vi "CS POLARIS BME DG.ProcCases.vi"(0 "i ref in":refnum<vi>, 1 "selector":string, 2 "Data":T1, 3 "call cluster":T2={"Object"="", "Selector"="", "CallType"=enum."synchronous", "Async Object"="", "Async Selector"="", "Data Descriptor"="", "Data"=[], "Error #"=0, "Expire"=0}, 5 "error in (no error)":errorcluster) -> (14 "i ref out":refnum<vi>, 17 "answer cluster":T2={"Object"="", "Selector"="", "CallType"=enum."synchronous", "Async Object"="", "Async Selector"="", "Data Descriptor"="", "Data"=[], "Error #"=0, "Expire"=0}, 19 "error out":errorcluster)   [LabVIEW 2009, in "CS POLARIS BME DG.lvlib"]
doc: "This method is called by a process from within the default case in the event loop. The methods of a class that are linked to events will be called from THIS method. Add your code here."
uses:
  CS POLARIS BME DG.lvlib
  CSCore/CSSystem/CoreDefs/CoreDefs.call_type.ctl
  CSCore/BaseProcess/BaseProcess.descriptor string definition.ctl
  CSCore/CSSystem/CoreDefs/CoreDefs.rawDataType.ctl
  CSCore/CSSystem/CoreLib/CoreLib.byte array 2 string.vi
  DG Classes/BME_DG_System/ControlLevel.ctl
  DG Classes/BME_DG_System/BME_DG_System.lvclass
  CSCore/CSSystem/CoreLib/CoreLib.byte array 2 int.vi
  DG Classes/BME_DG_Chnl/BME_DG_Chnl.lvclass
  CSCore/CSSystem/CoreLib/CoreLib.double 2 byte array.vi
  CSCore/CSSystem/CoreLib/CoreLib.string 2 byte array.vi
  CSCore/CSSystem/CoreLib/CoreLib.lvlib
  CSCore/BaseProcess/BaseProcess.lvlib
  CSApplicationBaseClasses/DeviceBase/DeviceBase.lvlib
  lib.lib/UtilityLib/UtilityLib.lvlib
  lib.lib/DimLVEvent/LVDimInterface/LVDimInterface.lvlib
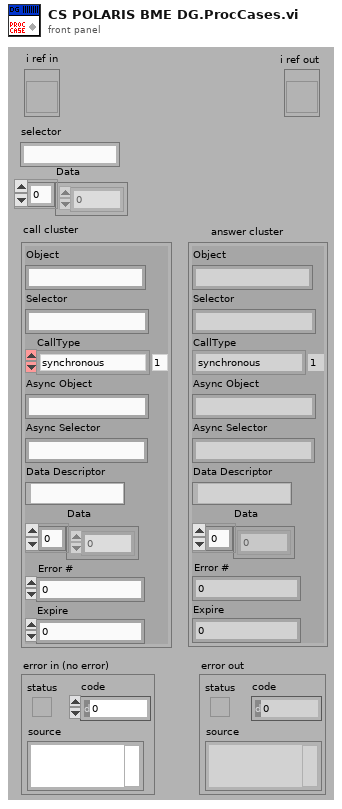
[diagram p1: front panel]
types:
  T1 = typedef "CoreDefs.rawDataType.ctl" = i8[]
  T2 = typedef "CoreDefs.call_type.ctl" = cluster{"Object":string, "Selector":string, "CallType":enum16{"simple", "synchronous", "asynchronous"}, "Async Object":string, "Async Selector":string, "Data Descriptor":T3, "Data":T1, "Error #":i32, "Expire":u32}
  T3 = typedef "BaseProcess.lvlib/BaseProcess.descriptor string definition.ctl" = string
  T4 = typedef "POLARIS BME DG.lvlib/BME_DG_System.lvclass/ControlLevel.ctl" = enum16{"Simple", "Expert", "Unknown"}
  T5 = typedef "POLARIS BME DG.lvlib/Chnl Settings Complete.ctl" = cluster{"Channel Name":string, "ChnParameter":T6, "DelayFormula":string, "OutputModulo":i32, "Go and Done Signal":T7, "G08_Chnl_Settings":T9}
  T6 = typedef "POLARIS BME DG.lvlib/ChnlSettings.ctl" = cluster{" Delay (µs)":dbl, "On?":bool, "PositiveVoltage?":bool, "50OhmTerminated? ":bool, "25OhmOutput?":bool}
  T7 = typedef "POLARIS BME DG.lvlib/Go_Done_Chnl_Settings.ctl" = cluster{"Go Signal":T8, "Done Signal":u32}
  T8 = typedef "POLARIS BME DG.lvlib/GoSignalBits.ctl" = u32
  T9 = typedef "POLARIS BME DG.lvlib/SG08_Chnl_Settings.ctl" = cluster{"Pulse Width (µs)":dbl, "Output Offset":u32, "Disconnect (E,F)":bool, "Onto MsBus (E,F)":bool, "Input Positive (E,F)":bool}
  T10 = typedef "CS POLARIS BME DG.lvlib/CS POLARIS BME DG.i attribute.ctl" = cluster{"DIMLockedBy":i32, "DG_System":refnum<queue>, "UpdateTasks":refnum<queue>, "SaveEachParamChng":bool, "SaveAtShutdown":bool, "DIMSecTillComShot":i32}
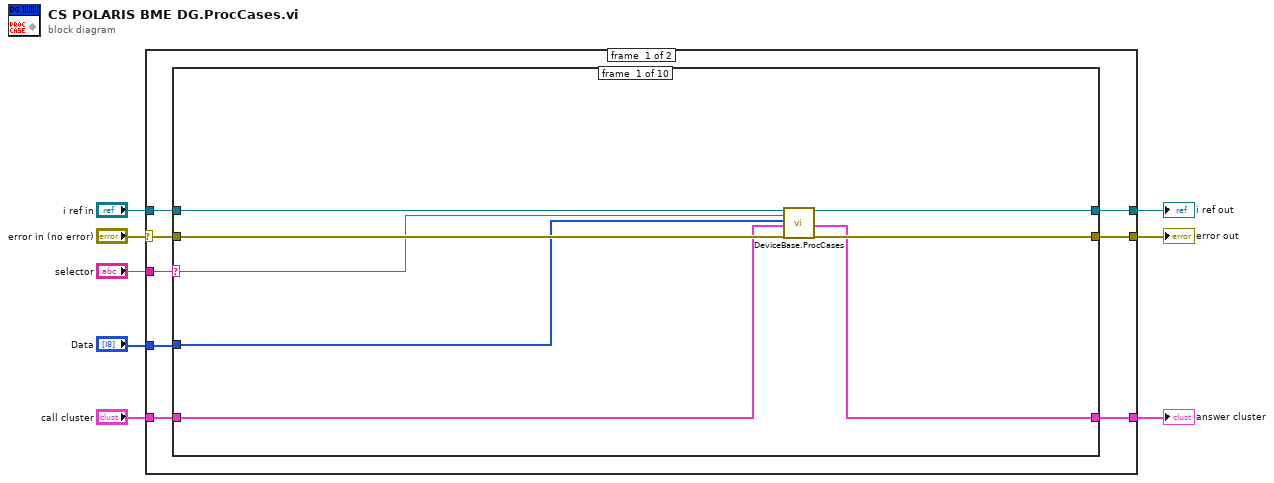
[diagram p0: block diagram]
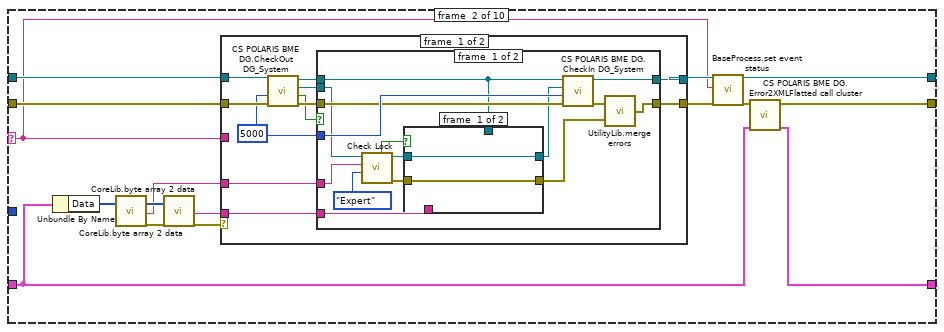
[diagram p2: hidden frame]
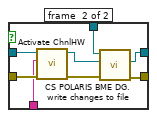
[diagram p3: hidden frame]
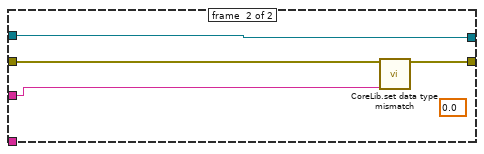
[diagram p5: hidden frame]
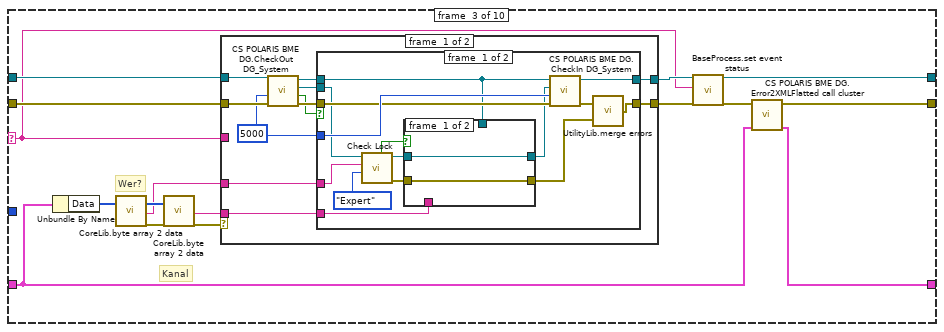
[diagram p6: hidden frame]
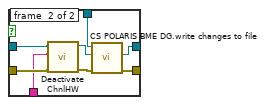
[diagram p7: hidden frame]
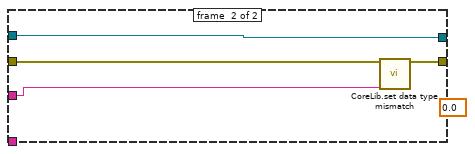
[diagram p9: hidden frame]
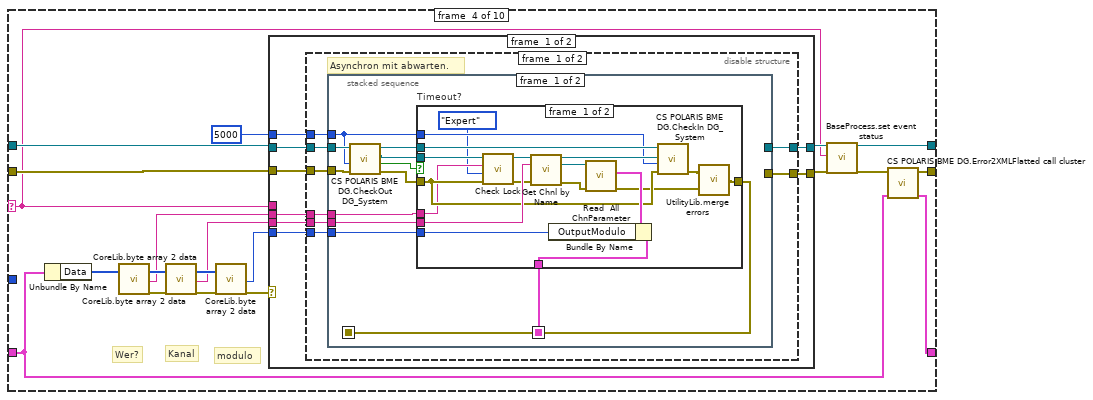
[diagram p10: hidden frame]
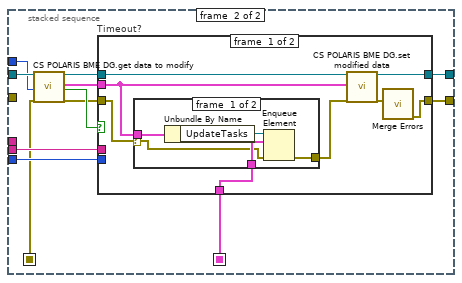
[diagram p12: hidden frame]
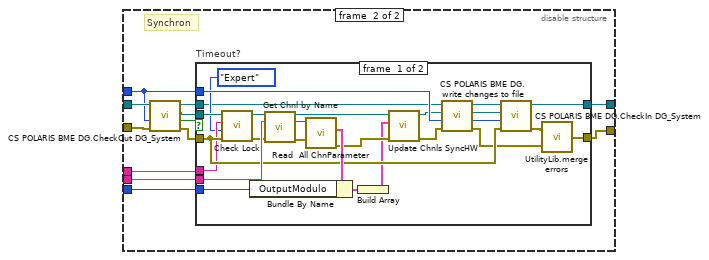
[diagram p15: hidden frame]
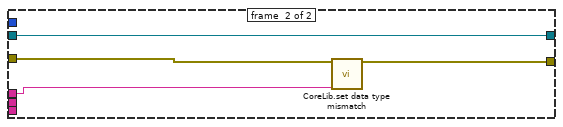
[diagram p17: hidden frame]
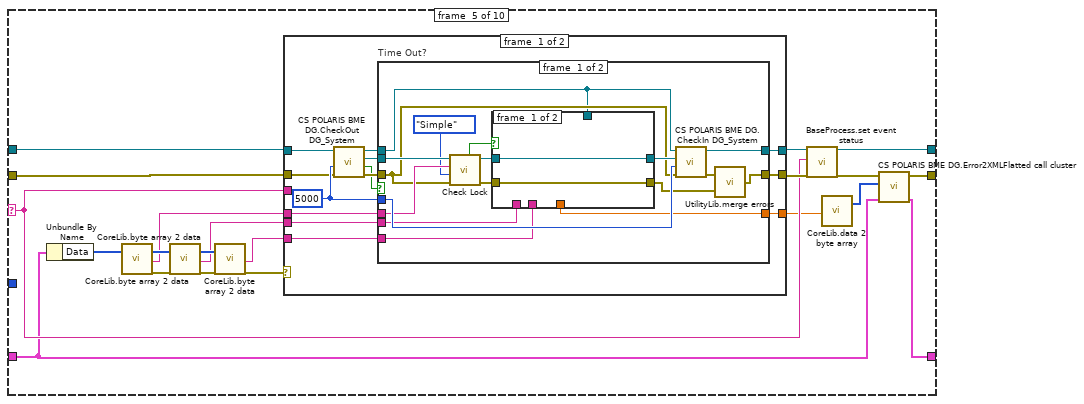
[diagram p18: hidden frame]
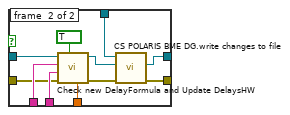
[diagram p19: hidden frame]
diagram:
  n1 = case shown="No Error" "error in (no error)" {
    selector: "error in (no error)" -> [w9 w596]
    tunnel: "selector" -> [w16 _]
    tunnel: [w15 w597] -> w7
    tunnel: "Data" -> [w14 _]
    tunnel: "call cluster" -> [w13 w597]
    tunnel: "i ref in" -> [w12 w598]
    tunnel: [w11 w598] -> w3
    tunnel: [w10 w596] -> w2
    frame #0 {
      n2 = case shown="\"SetDelayFormula\"" w16 {
        selector: w16 -> [w19 w36 w94 w156 w295 w361 w412 w462 w517 w562]
        tunnel: w14 -> [w17 _ _ _ _ _ _ _ _ _]
        tunnel: w12 -> [w18 w40 w98 w160 w299 w365 w416 w466 w521 w565]
        tunnel: [w24 w35 w93 w155 w294 w360 w411 w461 w516 w561] -> w11
        tunnel: w13 -> [w20 w30 w88 w146 w286 w351 w406 w455 w511 w558]
        tunnel: [w21 w29 w87 w147 w285 w350 w405 w454 w510 w557] -> w15
        tunnel: w9 -> [w23 w39 w97 w159 w298 w364 w415 w465 w520 w555]
        tunnel: [w22 w31 w89 w148 w287 w352 w407 w456 w512 w559] -> w10
        frame #0 {
          # "In the default case, always call the ProcCase method of the parent class"
          n3 = call "DeviceBase.ProcCases.vi"("i ref in"=w18, "selector"=w19, "Data"=w17, "call cluster"=w20, "error in (no error)"=w23) -> ("i ref out"=w24:refnum<vi>, "answer cluster"=w21:T2, "error out"=w22:errorcluster)  [unwired: 12 in]
        }
        frame #1 {
          # "This is just an example. On how to use this VI. The names of the selector should be identical to the name of the corresponding event. Inside the false case, place the method you want to call."
          n4 = Unbundle By Name(w30) -> ("Data"=w27:T1)
          n5 = call-poly "CoreLib.byte array 2 data.vi"("byteArray"=w27) -> ("byteArray out"=w28:T1, "string"=w25:string, "error out"=w26:errorcluster)  [unwired: 16 in]
          n6 = call-poly "CoreLib.byte array 2 data.vi"("byteArray"=w28, "error in (no error)"=w26) -> ("string"=w33:string, "error out"=w34:errorcluster)  [unwired: 15 in, 1 out]
          n7 = case shown="No Error" w34 {
            tunnel: [w46 w82] -> w38
            tunnel: w40 -> [w51 w82]
            tunnel: w39 -> [w50 w81]
            tunnel: [w44 w80] -> w37
            tunnel: w36 -> [_ w79]
            tunnel: w33 -> [w42 _]
            tunnel: w25 -> [w41 _]
            frame #0 {
              w43 = 5000 ("timeout in ms (-1)")
              n8 = call "CS POLARIS BME DG.CheckOut DG_System.vi"("error IO"=w50, "timeout in ms (-1)"=w43, "i ref in"=w51) -> ("error out"=w48:errorcluster, "Q timed out"=w47:bool, "BME_DG_System out"=w49:refnum<class "BME_DG_System.lvclass">, "i ref out"=w45:refnum<vi>)  [unwired: 5 in]
              n9 = case shown="False" w47 {
                tunnel: w49 -> [w57 _]
                tunnel: w48 -> [w64 w78]
                tunnel: [w62 w78] -> w44
                tunnel: [w66 w77] -> w46
                tunnel: w45 -> [w52 w77]
                tunnel: w43 -> [w65 _]
                tunnel: w42 -> [w54 _]
                tunnel: w41 -> [w53 _]
                frame #0 {
                  n10 = call-dynamic "Check Lock.vi"("Control level"=ControlLevel."Expert", "Name"=w53, "BME_DG_System in"=w57) -> ("error out"=w61:errorcluster, "BME_DG_System out"=w60:refnum<class "BME_DG_System.lvclass">, "Ok?"=w58:bool)  [unwired: 4 in, 2 out]
                  n11 = case shown="True" w58 {
                    tunnel: [w68 w70] -> w55
                    tunnel: w54 -> [_ w74]
                    tunnel: [w67 w69] -> w56
                    tunnel: w61 -> [w67 w75]
                    tunnel: w60 -> [w68 w76]
                    tunnel: w52 -> [_ w73]
                    frame #0 {
                    }
                    frame #1 {
                      n12 = call "Activate ChnlHW.vi"("error in (no error)"=w75, "ChnlName"=w74, "BME_DG_System in"=w76) -> ("error out"=w71:errorcluster, "BME_DG_System out"=w72:refnum<class "BME_DG_System.lvclass">)  [unwired: 7 in]
                      n13 = call "CS POLARIS BME DG.write changes to file.vi"("error in"=w71, "BME_DG_System in"=w72, "i ref in"=w73) -> ("error in"=w69:errorcluster, "BME_DG_System out"=w70:refnum<class "BME_DG_System.lvclass">)  [unwired: 5 in, 1 out]
                    }
                  }
                  n14 = call "CS POLARIS BME DG.CheckIn DG_System.vi"("error in"=w64, "timeout in ms (-1)"=w65, "BME_DG_System"=w55, "i ref in"=w52) -> ("error in"=w63:errorcluster, "i ref out"=w66:refnum<vi>)  [unwired: 5 in]
                  n15 = call "UtilityLib.merge errors.vi"("error2 (no error)"=w56, "error1 (no error)"=w63) -> ("error out"=w62:errorcluster)
                }
                frame #1 {
                }
              }
            }
            frame #1 {
              (unwired) 0.0
              n16 = call "CoreLib.set data type mismatch.vi"("error in (no error)"=w81, "error source"=w79) -> ("error out"=w80:errorcluster)  [unwired: 17 in]
            }
          }
          n17 = call "BaseProcess.set event status.vi"("i ref in"=w38, "EventStatus"=w36, "error in (no error)"=w37) -> ("i ref out"=w35:refnum<vi>, "error out"=w32:errorcluster)  [unwired: 14 in, 1 out]
          n18 = call "CS POLARIS BME DG.Error2XMLFlatted call cluster.vi"("call cluster in"=w30, "error in"=w32) -> ("call cluster out"=w29:T2, "error out"=w31:errorcluster)  [unwired: 8 in]
        }
        frame #2 {
          # "Kanal"
          # "Wer?"
          # "This is just an example. On how to use this VI. The names of the selector should be identical to the name of the corresponding event. Inside the false case, place the method you want to call."
          n19 = Unbundle By Name(w88) -> ("Data"=w85:T1)
          n20 = call-poly "CoreLib.byte array 2 data.vi"("byteArray"=w85) -> ("byteArray out"=w86:T1, "string"=w83:string, "error out"=w84:errorcluster)  [unwired: 16 in]
          n21 = call-poly "CoreLib.byte array 2 data.vi"("byteArray"=w86, "error in (no error)"=w84) -> ("string"=w91:string, "error out"=w92:errorcluster)  [unwired: 15 in, 1 out]
          n22 = case shown="No Error" w92 {
            tunnel: [w104 w140] -> w96
            tunnel: w98 -> [w109 w140]
            tunnel: w97 -> [w108 w139]
            tunnel: [w102 w138] -> w95
            tunnel: w94 -> [_ w137]
            tunnel: w91 -> [w100 _]
            tunnel: w83 -> [w99 _]
            frame #0 {
              w101 = 5000 ("timeout in ms (-1)")
              n23 = call "CS POLARIS BME DG.CheckOut DG_System.vi"("error IO"=w108, "timeout in ms (-1)"=w101, "i ref in"=w109) -> ("error out"=w106:errorcluster, "Q timed out"=w105:bool, "BME_DG_System out"=w107:refnum<class "BME_DG_System.lvclass">, "i ref out"=w103:refnum<vi>)  [unwired: 5 in]
              n24 = case shown="False" w105 {
                tunnel: w107 -> [w115 _]
                tunnel: w106 -> [w122 w136]
                tunnel: [w120 w136] -> w102
                tunnel: [w124 w135] -> w104
                tunnel: w103 -> [w110 w135]
                tunnel: w101 -> [w123 _]
                tunnel: w100 -> [w112 _]
                tunnel: w99 -> [w111 _]
                frame #0 {
                  n25 = call-dynamic "Check Lock.vi"("Control level"=ControlLevel."Expert", "Name"=w111, "BME_DG_System in"=w115) -> ("error out"=w119:errorcluster, "BME_DG_System out"=w118:refnum<class "BME_DG_System.lvclass">, "Ok?"=w116:bool)  [unwired: 4 in, 2 out]
                  n26 = case shown="True" w116 {
                    tunnel: [w126 w128] -> w113
                    tunnel: w112 -> [_ w132]
                    tunnel: [w125 w127] -> w114
                    tunnel: w119 -> [w125 w133]
                    tunnel: w118 -> [w126 w134]
                    tunnel: w110 -> [_ w131]
                    frame #0 {
                    }
                    frame #1 {
                      n27 = call "Deactivate ChnlHW.vi"("error in (no error)"=w133, "ChnlName"=w132, "BME_DG_System in"=w134) -> ("error out"=w129:errorcluster, "BME_DG_System out"=w130:refnum<class "BME_DG_System.lvclass">)  [unwired: 7 in]
                      n28 = call "CS POLARIS BME DG.write changes to file.vi"("error in"=w129, "BME_DG_System in"=w130, "i ref in"=w131) -> ("error in"=w127:errorcluster, "BME_DG_System out"=w128:refnum<class "BME_DG_System.lvclass">)  [unwired: 5 in, 1 out]
                    }
                  }
                  n29 = call "CS POLARIS BME DG.CheckIn DG_System.vi"("error in"=w122, "timeout in ms (-1)"=w123, "BME_DG_System"=w113, "i ref in"=w110) -> ("error in"=w121:errorcluster, "i ref out"=w124:refnum<vi>)  [unwired: 5 in]
                  n30 = call "UtilityLib.merge errors.vi"("error2 (no error)"=w114, "error1 (no error)"=w121) -> ("error out"=w120:errorcluster)
                }
                frame #1 {
                }
              }
            }
            frame #1 {
              (unwired) 0.0
              n31 = call "CoreLib.set data type mismatch.vi"("error in (no error)"=w139, "error source"=w137) -> ("error out"=w138:errorcluster)  [unwired: 17 in]
            }
          }
          n32 = call "BaseProcess.set event status.vi"("i ref in"=w96, "EventStatus"=w94, "error in (no error)"=w95) -> ("i ref out"=w93:refnum<vi>, "error out"=w90:errorcluster)  [unwired: 14 in, 1 out]
          n33 = call "CS POLARIS BME DG.Error2XMLFlatted call cluster.vi"("call cluster in"=w88, "error in"=w90) -> ("call cluster out"=w87:T2, "error out"=w89:errorcluster)  [unwired: 8 in]
        }
        frame #3 {
          # "modulo"
          # "Kanal"
          # "Wer?"
          n34 = Unbundle By Name(w146) -> ("Data"=w143:T1)
          n35 = call-poly "CoreLib.byte array 2 data.vi"("byteArray"=w143) -> ("byteArray out"=w142:T1, "string"=w141:string, "error out"=w144:errorcluster)  [unwired: 16 in]
          n36 = call-poly "CoreLib.byte array 2 data.vi"("byteArray"=w142, "error in (no error)"=w144) -> ("byteArray out"=w153:T1, "string"=w151:string, "error out"=w154:errorcluster)  [unwired: 15 in]
          n37 = call-poly "CoreLib.byte array 2 data.vi"("byteArray"=w153, "error in (no error)"=w154) -> ("i32"=w150:i32, "error out"=w152:errorcluster)  [unwired: 15 in, 1 out]
          n38 = case shown="No Error" w152 {
            tunnel: [w167 w278] -> w158
            tunnel: w160 -> [w168 w278]
            tunnel: w159 -> [w165 w277]
            tunnel: [w166 w276] -> w157
            tunnel: w150 -> [w163 _]
            tunnel: w156 -> [_ w275]
            tunnel: w151 -> [w164 _]
            tunnel: 5000 -> [w162 _]
            tunnel: w141 -> [w161 _]
            frame #0 {
              n39 = disable-structure shown="Enabled" {
                disable-tunnel: w168 -> [w176 w247]
                disable-tunnel: [w175 w246] -> w167
                disable-tunnel: [w174 w245] -> w166
                disable-tunnel: w165 -> [w173 w244]
                disable-tunnel: w164 -> [w172 w243]
                disable-tunnel: w163 -> [w171 w242]
                disable-tunnel: w162 -> [w170 w241]
                disable-tunnel: w161 -> [w169 w240]
                frame #0 {
                  # "Asynchron mit abwarten."
                  n40 = stacked-sequence {
                    seq-local: [w178 _] -> [_ w211]
                    seq-local: [w177 _] -> [_ w209]
                    tunnel: w176 -> [w186 w219]
                    tunnel: [_ w210] -> w175
                    tunnel: [_ w215] -> w174
                    tunnel: w173 -> [w184 _]
                    tunnel: w172 -> [w188 w213]
                    tunnel: w171 -> [w187 w212]
                    tunnel: w170 -> [w180 w208]
                    tunnel: w169 -> [w179 _]
                    frame #0 {
                      n41 = call "CS POLARIS BME DG.CheckOut DG_System.vi"("error IO"=w184, "timeout in ms (-1)"=w180, "i ref in"=w186) -> ("error out"=w183:errorcluster, "Q timed out"=w181:bool, "BME_DG_System out"=w182:refnum<class "BME_DG_System.lvclass">, "i ref out"=w185:refnum<vi>)  [unwired: 5 in]
                      n42 = case "Timeout?" shown="False" w181 {
                        tunnel: w185 -> [w206 _]
                        tunnel: w182 -> [w197 _]
                        tunnel: [w190 w207] -> w178
                        tunnel: w183 -> [w198 w207]
                        tunnel: w188 -> [w200 _]
                        tunnel: w187 -> [w201 _]
                        tunnel: w180 -> [w199 _]
                        tunnel: w179 -> [w194 _]
                        tunnel: [w189 _] -> w177
                        frame #0 {
                          n43 = call-dynamic "Check Lock.vi"("error in (no error)"=w198, "Control level"=ControlLevel."Expert", "Name"=w194, "BME_DG_System in"=w197) -> ("error out"=w195:errorcluster, "BME_DG_System out"=w196:refnum<class "BME_DG_System.lvclass">)  [unwired: 3 in, 3 out]
                          n44 = call "Get Chnl by Name.vi"("BME_DG_System in"=w196, "Chnl Name"=w200, "error in (no error)"=w195) -> ("BME_DG_System out"=w204:refnum<class "BME_DG_System.lvclass">, "BME_DG_Chnl"=w205:refnum<class "BME_DG_Chnl.lvclass">, "error out"=w203:errorcluster)  [unwired: 7 in, 3 out]
                          n45 = call-dynamic "Read  All ChnParameter.vi"("error in (no error)"=w203, "BME_DG_Chnl in"=w205) -> ("error out"=w191:errorcluster, "ChnlParam"=w202:T5)  [unwired: 7 in, 1 out]
                          n46 = Bundle By Name(cluster=w202, "OutputModulo"=w201) -> (w189:T5)
                          n47 = call "CS POLARIS BME DG.CheckIn DG_System.vi"("error in"=w198, "timeout in ms (-1)"=w199, "BME_DG_System"=w204, "i ref in"=w206) -> ("error in"=w192:errorcluster)  [unwired: 5 in, 1 out]
                          n48 = call "UtilityLib.merge errors.vi"("error2 (no error)"=w191, "error1 (no error)"=w192) -> ("error out"=w190:errorcluster)
                        }
                        frame #1 {
                        }
                      }
                    }
                    frame #1 {
                      n49 = call "CS POLARIS BME DG.get data to modify.vi"("i ref in"=w219, "ms timeout (10000)"=w208, "error in (no error)"=w211) -> ("i ref out"=w218:refnum<vi>, "i attribute"=w216:T10, "timed out"=w217:bool, "error out"=w214:errorcluster)  [unwired: 13 in]
                      n50 = case "Timeout?" shown="False" w217 {
                        tunnel: w218 -> [w227 w234]
                        tunnel: [w226 w234] -> w210
                        tunnel: w216 -> [w224 _]
                        tunnel: [w222 w235] -> w215
                        tunnel: w214 -> [w221 w235]
                        tunnel: w213 -> [_ _]
                        tunnel: w212 -> [_ _]
                        tunnel: w209 -> [w223 _]
                        frame #0 {
                          n51 = case shown="No Error" w221 {
                            selector: w221 -> [w228 w233]
                            tunnel: w224 -> [w232 _]
                            tunnel: w223 -> [w230 _]
                            tunnel: [w229 w233] -> w220
                            frame #0 {
                              n52 = Unbundle By Name(w232) -> ("UpdateTasks"=w231:refnum<queue>)
                              n53 = Enqueue Element(queue=w231, element=w230, error in (no error)=w228) -> (error out=w229:errorcluster)  [unwired: 1 in, 2 out]
                            }
                            frame #1 {
                            }
                          }
                          n54 = call "CS POLARIS BME DG.set modified data.vi"("i ref in"=w227, "i attribute"=w224, "error in (no error)"=w220) -> ("i ref out"=w226:refnum<vi>, "error out"=w225:errorcluster)  [unwired: 15 in]
                          n55 = call <vilib>:"Merge Errors.vi"("error in 2 (no error)"=w225) -> ("error out"=w222:errorcluster)  [unwired: 6 in]
                        }
                        frame #1 {
                        }
                      }
                    }
                  }
                }
                frame #1 {
                  # "Synchron"
                  n56 = call "CS POLARIS BME DG.CheckOut DG_System.vi"("error IO"=w244, "timeout in ms (-1)"=w241, "i ref in"=w247) -> ("error out"=w238:errorcluster, "Q timed out"=w236:bool, "BME_DG_System out"=w237:refnum<class "BME_DG_System.lvclass">, "i ref out"=w239:refnum<vi>)  [unwired: 5 in]
                  n57 = case "Timeout?" shown="False" w236 {
                    tunnel: w239 -> [w253 w273]
                    tunnel: w237 -> [w265 _]
                    tunnel: [w259 w274] -> w245
                    tunnel: w238 -> [w266 w274]
                    tunnel: w243 -> [w268 _]
                    tunnel: w242 -> [w269 _]
                    tunnel: w241 -> [w267 _]
                    tunnel: w240 -> [w262 _]
                    tunnel: [w254 w273] -> w246
                    frame #0 {
                      n58 = call-dynamic "Check Lock.vi"("error in (no error)"=w266, "Control level"=ControlLevel."Expert", "Name"=w262, "BME_DG_System in"=w265) -> ("error out"=w263:errorcluster, "BME_DG_System out"=w264:refnum<class "BME_DG_System.lvclass">)  [unwired: 3 in, 3 out]
                      n59 = call "Get Chnl by Name.vi"("BME_DG_System in"=w264, "Chnl Name"=w268, "error in (no error)"=w263) -> ("BME_DG_System out"=w258:refnum<class "BME_DG_System.lvclass">, "BME_DG_Chnl"=w272:refnum<class "BME_DG_Chnl.lvclass">, "error out"=w271:errorcluster)  [unwired: 7 in, 3 out]
                      n60 = call-dynamic "Read  All ChnParameter.vi"("error in (no error)"=w271, "BME_DG_Chnl in"=w272) -> ("error out"=w257:errorcluster, "ChnlParam"=w270:T5)  [unwired: 7 in, 1 out]
                      n61 = Bundle By Name(cluster=w270, "OutputModulo"=w269) -> (w256:T5)
                      n62 = Build Array(w256) -> (w255:T5[])
                      n63 = call "Update Chnls SyncHW.vi"("error in (no error)"=w257, "ChnlSettings"=w255, "BME_DG_System in"=w258) -> ("error out"=w249:errorcluster, "BME_DG_System out"=w251:refnum<class "BME_DG_System.lvclass">)  [unwired: 6 in, 1 out]
                      n64 = call "CS POLARIS BME DG.write changes to file.vi"("error in"=w249, "BME_DG_System in"=w251, "i ref in"=w253) -> ("error in"=w248:errorcluster, "BME_DG_System out"=w250:refnum<class "BME_DG_System.lvclass">, "i ref out"=w252:refnum<vi>)  [unwired: 5 in]
                      n65 = call "CS POLARIS BME DG.CheckIn DG_System.vi"("error in"=w266, "timeout in ms (-1)"=w267, "BME_DG_System"=w250, "i ref in"=w252) -> ("error in"=w260:errorcluster, "i ref out"=w254:refnum<vi>)  [unwired: 5 in]
                      n66 = call "UtilityLib.merge errors.vi"("error2 (no error)"=w248, "error1 (no error)"=w260) -> ("error out"=w259:errorcluster)
                    }
                    frame #1 {
                    }
                  }
                }
              }
            }
            frame #1 {
              n67 = call "CoreLib.set data type mismatch.vi"("error in (no error)"=w277, "error source"=w275) -> ("error out"=w276:errorcluster)  [unwired: 17 in]
            }
          }
          n68 = call "BaseProcess.set event status.vi"("i ref in"=w158, "EventStatus"=w156, "error in (no error)"=w157) -> ("i ref out"=w155:refnum<vi>, "error out"=w149:errorcluster)  [unwired: 14 in, 1 out]
          n69 = call "CS POLARIS BME DG.Error2XMLFlatted call cluster.vi"("call cluster in"=w146, "error in"=w149) -> ("call cluster out"=w147:T2, "error out"=w148:errorcluster)  [unwired: 8 in]
        }
        frame #4 {
          # "This is just an example. On how to use this VI. The names of the selector should be identical to the name of the corresponding event. Inside the false case, place the method you want to call."
          n70 = Unbundle By Name(w286) -> ("Data"=w284:T1)
          n71 = call-poly "CoreLib.byte array 2 data.vi"("byteArray"=w284) -> ("byteArray out"=w283:T1, "string"=w281:string, "error out"=w282:errorcluster)  [unwired: 16 in]
          n72 = call-poly "CoreLib.byte array 2 data.vi"("byteArray"=w283, "error in (no error)"=w282) -> ("byteArray out"=w292:T1, "string"=w290:string, "error out"=w293:errorcluster)  [unwired: 15 in]
          n73 = call-poly "CoreLib.byte array 2 data.vi"("byteArray"=w292, "error in (no error)"=w293) -> ("string"=w289:string, "error out"=w291:errorcluster)  [unwired: 15 in, 1 out]
          n74 = case shown="No Error" w291 {
            tunnel: [w305 w348] -> w297
            tunnel: w299 -> [w307 w348]
            tunnel: w298 -> [w306 w347]
            tunnel: [w304 w346] -> w296
            tunnel: w289 -> [w302 _]
            tunnel: w295 -> [_ w345]
            tunnel: w290 -> [w303 _]
            tunnel: w281 -> [w301 _]
            tunnel: [w300 _] -> w279
            frame #0 {
              w308 = 5000 ("timeout in ms (-1)")
              n75 = call "CS POLARIS BME DG.CheckOut DG_System.vi"("error IO"=w306, "timeout in ms (-1)"=w308, "i ref in"=w307) -> ("error out"=w311:errorcluster, "Q timed out"=w310:bool, "BME_DG_System out"=w312:refnum<class "BME_DG_System.lvclass">, "i ref out"=w309:refnum<vi>)  [unwired: 5 in]
              n76 = case "Time Out?" shown="False" w310 {
                tunnel: w312 -> [w320 _]
                tunnel: w311 -> [w315 w344]
                tunnel: [w322 w344] -> w304
                tunnel: [w329 w343] -> w305
                tunnel: w309 -> [w314 w343]
                tunnel: w308 -> [w328 _]
                tunnel: w303 -> [w326 _]
                tunnel: w302 -> [w325 _]
                tunnel: w301 -> [w318 _]
                tunnel: [w313 _] -> w300
                frame #0 {
                  n77 = call-dynamic "Check Lock.vi"("error in (no error)"=w315, "Control level"=ControlLevel."Simple", "Name"=w318, "BME_DG_System in"=w320) -> ("error out"=w321:errorcluster, "BME_DG_System out"=w319:refnum<class "BME_DG_System.lvclass">, "Ok?"=w316:bool)  [unwired: 3 in, 2 out]
                  n78 = case shown="True" w316 {
                    tunnel: [w331 w334] -> w327
                    tunnel: w326 -> [_ w341]
                    tunnel: w325 -> [_ w340]
                    tunnel: [w330 w336] -> w323
                    tunnel: w321 -> [w330 w339]
                    tunnel: w319 -> [w331 w338]
                    tunnel: w314 -> [_ w333]
                    tunnel: [_ w332] -> w313
                    frame #0 {
                    }
                    frame #1 {
                      n79 = call "Check new DelayFormula and Update DelaysHW.vi"("Update HW?(false)"=TRUE ("Update HW"), "error in (no error)"=w339, "Delay Formula"=w340, "ChnlName"=w341, "BME_DG_System in"=w338) -> ("error out"=w337:errorcluster, "BME_DG_System out"=w335:refnum<class "BME_DG_System.lvclass">, "Abs. Delay"=w332:dbl)  [unwired: 3 in, 1 out]
                      n80 = call "CS POLARIS BME DG.write changes to file.vi"("error in"=w337, "BME_DG_System in"=w335, "i ref in"=w333) -> ("error in"=w336:errorcluster, "BME_DG_System out"=w334:refnum<class "BME_DG_System.lvclass">)  [unwired: 5 in, 1 out]
                    }
                  }
                  n81 = call "CS POLARIS BME DG.CheckIn DG_System.vi"("error in"=w315, "timeout in ms (-1)"=w328, "BME_DG_System"=w327, "i ref in"=w314) -> ("error in"=w324:errorcluster, "i ref out"=w329:refnum<vi>)  [unwired: 5 in]
                  n82 = call "UtilityLib.merge errors.vi"("error2 (no error)"=w323, "error1 (no error)"=w324) -> ("error out"=w322:errorcluster)
                }
                frame #1 {
                }
              }
            }
            frame #1 {
              n83 = call "CoreLib.set data type mismatch.vi"("error in (no error)"=w347, "error source"=w345) -> ("error out"=w346:errorcluster)  [unwired: 17 in]
            }
          }
          n84 = call "BaseProcess.set event status.vi"("i ref in"=w297, "EventStatus"=w295, "error in (no error)"=w296) -> ("i ref out"=w294:refnum<vi>, "error out"=w288:errorcluster)  [unwired: 14 in, 1 out]
          n85 = call-poly "CoreLib.data 2 byte array.vi"("f64"=w279) -> ("byteArray out"=w280:T1)  [unwired: 18 in]
          n86 = call "CS POLARIS BME DG.Error2XMLFlatted call cluster.vi"("call cluster in"=w286, "byteArray in"=w280, "error in"=w288) -> ("call cluster out"=w285:T2, "error out"=w287:errorcluster)  [unwired: 7 in]
        }
        frame #5 {
          # "Simple = 0\nExpert =1"
          # "Wer?"
          # "This is just an example. On how to use this VI. The names of the selector should be identical to the name of the corresponding event. Inside the false case, place the method you want to call."
          n87 = Unbundle By Name(w351) -> ("Data"=w359:T1)
          n88 = call-poly "CoreLib.byte array 2 data.vi"("byteArray"=w359) -> ("byteArray out"=w357:T1, "string"=w355:string, "error out"=w358:errorcluster)  [unwired: 16 in]
          n89 = call-poly "CoreLib.byte array 2 data.vi"("byteArray"=w357, "error in (no error)"=w358) -> ("i32"=w354:i32, "error out"=w356:errorcluster)  [unwired: 15 in, 1 out]
          n90 = case shown="No Error" w356 {
            tunnel: [w370 w401] -> w363
            tunnel: w365 -> [w372 w401]
            tunnel: w364 -> [w371 w400]
            tunnel: [w369 w399] -> w362
            tunnel: w354 -> [w367 _]
            tunnel: w361 -> [_ w398]
            tunnel: w355 -> [w368 _]
            tunnel: [w366 _] -> w349
            frame #0 {
              w373 = 5000 ("timeout in ms (-1)")
              n91 = call "CS POLARIS BME DG.CheckOut DG_System.vi"("error IO"=w371, "timeout in ms (-1)"=w373, "i ref in"=w372) -> ("error out"=w376:errorcluster, "Q timed out"=w375:bool, "BME_DG_System out"=w377:refnum<class "BME_DG_System.lvclass">, "i ref out"=w374:refnum<vi>)  [unwired: 5 in]
              n92 = case "Time Out?" shown="False" w375 {
                tunnel: w377 -> [w391 _]
                tunnel: w376 -> [w389 w397]
                tunnel: [w392 w397] -> w369
                tunnel: [w395 w396] -> w370
                tunnel: w374 -> [w384 w396]
                tunnel: w373 -> [w394 _]
                tunnel: w368 -> [w387 _]
                tunnel: w367 -> [w386 _]
                tunnel: [w385 _] -> w366
                frame #0 {
                  n93 = call "CS POLARIS BME DG.get i attribute.vi"("i ref in"=w384) -> ("i attribute"=w383:T10)  [unwired: 16 in, 2 out]
                  n94 = Unbundle By Name(w383) -> ("DIMLockedBy"=w382:i32)
                  n95 = call "RequestControl.vi"("error in (no error)"=w389, "level in"=w386, "who wants?"=w387, "BME_DG_System in"=w391) -> ("error out"=w388:errorcluster, "locked by out"=w379:string, "BME_DG_System out"=w390:refnum<class "BME_DG_System.lvclass">)  [unwired: 3 in, 2 out]
                  n96 = call "UtilityLib.align string.vi"("stringIn"=w379) -> ("stringOut"=w381:string, "error out"=w380:errorcluster)  [unwired: 17 in]
                  n97 = call "CS POLARIS BME DG.CheckIn DG_System.vi"("error in"=w389, "timeout in ms (-1)"=w394, "BME_DG_System"=w390, "i ref in"=w384) -> ("error in"=w393:errorcluster, "i ref out"=w395:refnum<vi>)  [unwired: 5 in]
                  n98 = call-poly "CoreLib.data 2 byte array.vi"("string"=w379) -> ("byteArray out"=w385:T1)  [unwired: 18 in]
                  n99 = call "LVDimInterface.dis_update_service.vi"("my_serviceID"=w382, "data"=w381, "error in (no error)"=w380) -> ("error out"=w378:errorcluster)  [unwired: 14 in, 2 out]
                  n100 = call "UtilityLib.merge errors.vi"("error2 (no error)"=w388, "error1 (no error)"=w393) -> ("error out"=w392:errorcluster)
                  n101 = call <vilib>:"Clear Errors.vi"("error in (no error)"=w378) -> ()  [unwired: 6 in, 1 out]
                }
                frame #1 {
                }
              }
            }
            frame #1 {
              n102 = call "CoreLib.set data type mismatch.vi"("error in (no error)"=w400, "error source"=w398) -> ("error out"=w399:errorcluster)  [unwired: 17 in]
            }
          }
          n103 = call "BaseProcess.set event status.vi"("i ref in"=w363, "EventStatus"=w361, "error in (no error)"=w362) -> ("i ref out"=w360:refnum<vi>, "error out"=w353:errorcluster)  [unwired: 14 in, 1 out]
          n104 = call "CS POLARIS BME DG.Error2XMLFlatted call cluster.vi"("call cluster in"=w351, "byteArray in"=w349, "error in"=w353) -> ("call cluster out"=w350:T2, "error out"=w352:errorcluster)  [unwired: 7 in]
        }
        frame #6 {
          # "Simple = 0\nExpert =1"
          # "Wer?"
          # "This is just an example. On how to use this VI. The names of the selector should be identical to the name of the corresponding event. Inside the false case, place the method you want to call."
          n105 = Unbundle By Name(w406) -> ("Data"=w410:T1)
          n106 = call-poly "CoreLib.byte array 2 data.vi"("byteArray"=w410) -> ("string"=w409:string, "error out"=w403:errorcluster)  [unwired: 16 in, 1 out]
          n107 = case shown="No Error" w403 {
            tunnel: [w421 w452] -> w414
            tunnel: w416 -> [w423 w452]
            tunnel: w415 -> [w422 w451]
            tunnel: [w420 w450] -> w413
            tunnel: ControlLevel."Simple" ("Control level") -> [w418 _]
            tunnel: w412 -> [_ w449]
            tunnel: w409 -> [w419 _]
            tunnel: [w417 _] -> w404
            frame #0 {
              w424 = 5000 ("timeout in ms (-1)")
              n108 = call "CS POLARIS BME DG.CheckOut DG_System.vi"("error IO"=w422, "timeout in ms (-1)"=w424, "i ref in"=w423) -> ("error out"=w427:errorcluster, "Q timed out"=w426:bool, "BME_DG_System out"=w428:refnum<class "BME_DG_System.lvclass">, "i ref out"=w425:refnum<vi>)  [unwired: 5 in]
              n109 = case "Time Out?" shown="False" w426 {
                tunnel: w428 -> [w435 _]
                tunnel: w427 -> [w434 w448]
                tunnel: [w443 w448] -> w420
                tunnel: [w446 w447] -> w421
                tunnel: w425 -> [w441 w447]
                tunnel: w424 -> [w445 _]
                tunnel: w419 -> [w432 _]
                tunnel: w418 -> [w429 _]
                tunnel: [w442 _] -> w417
                frame #0 {
                  n110 = call "CS POLARIS BME DG.get i attribute.vi"("i ref in"=w441) -> ("i attribute"=w440:T10)  [unwired: 16 in, 2 out]
                  n111 = Unbundle By Name(w440) -> ("DIMLockedBy"=w439:i32)
                  n112 = call "RequestControlForced.vi"("error in (no error)"=w434, "level in"=w429, "locked by"=w432, "BME_DG_System in"=w435) -> ("error out"=w433:errorcluster, "locked by out"=w430:string, "BME_DG_System out"=w431:refnum<class "BME_DG_System.lvclass">)  [unwired: 3 in, 2 out]
                  n113 = call "UtilityLib.align string.vi"("stringIn"=w430) -> ("stringOut"=w438:string, "error out"=w437:errorcluster)  [unwired: 17 in]
                  n114 = call "CS POLARIS BME DG.CheckIn DG_System.vi"("error in"=w434, "timeout in ms (-1)"=w445, "BME_DG_System"=w431, "i ref in"=w441) -> ("error in"=w444:errorcluster, "i ref out"=w446:refnum<vi>)  [unwired: 5 in]
                  n115 = call "LVDimInterface.dis_update_service.vi"("my_serviceID"=w439, "data"=w438, "error in (no error)"=w437) -> ("error out"=w436:errorcluster)  [unwired: 14 in, 2 out]
                  n116 = call-poly "CoreLib.data 2 byte array.vi"("string"=w430) -> ("byteArray out"=w442:T1)  [unwired: 18 in]
                  n117 = call "UtilityLib.merge errors.vi"("error2 (no error)"=w433, "error1 (no error)"=w444) -> ("error out"=w443:errorcluster)
                  n118 = call <vilib>:"Clear Errors.vi"("error in (no error)"=w436) -> ()  [unwired: 6 in, 1 out]
                }
                frame #1 {
                }
              }
            }
            frame #1 {
              n119 = call "CoreLib.set data type mismatch.vi"("error in (no error)"=w451, "error source"=w449) -> ("error out"=w450:errorcluster)  [unwired: 17 in]
            }
          }
          n120 = call "BaseProcess.set event status.vi"("i ref in"=w414, "EventStatus"=w412, "error in (no error)"=w413) -> ("i ref out"=w411:refnum<vi>, "error out"=w408:errorcluster)  [unwired: 14 in, 1 out]
          n121 = call "CS POLARIS BME DG.Error2XMLFlatted call cluster.vi"("call cluster in"=w406, "byteArray in"=w404, "error in"=w408) -> ("call cluster out"=w405:T2, "error out"=w407:errorcluster)  [unwired: 7 in]
        }
        frame #7 {
          # "This is just an example. On how to use this VI. The names of the selector should be identical to the name of the corresponding event. Inside the false case, place the method you want to call."
          n122 = Unbundle By Name(w455) -> ("Data"=w460:T1)
          n123 = call-poly "CoreLib.byte array 2 data.vi"("byteArray"=w460) -> ("string"=w458:string, "error out"=w459:errorcluster)  [unwired: 16 in, 1 out]
          n124 = case shown="No Error" w459 {
            tunnel: [w470 w501] -> w464
            tunnel: w466 -> [w472 w501]
            tunnel: w465 -> [w471 w500]
            tunnel: [w469 w499] -> w463
            tunnel: w462 -> [_ w498]
            tunnel: w458 -> [w468 _]
            tunnel: [w467 _] -> w453
            frame #0 {
              w473 = 5000 ("timeout in ms (-1)")
              n125 = call "CS POLARIS BME DG.CheckOut DG_System.vi"("error IO"=w471, "timeout in ms (-1)"=w473, "i ref in"=w472) -> ("error out"=w476:errorcluster, "Q timed out"=w475:bool, "BME_DG_System out"=w477:refnum<class "BME_DG_System.lvclass">, "i ref out"=w474:refnum<vi>)  [unwired: 5 in]
              n126 = case "Time Out?" shown="False" w475 {
                tunnel: w477 -> [w491 _]
                tunnel: w476 -> [w489 w497]
                tunnel: [w492 w497] -> w469
                tunnel: [w495 w496] -> w470
                tunnel: w474 -> [w480 w496]
                tunnel: w473 -> [w494 _]
                tunnel: w468 -> [w487 _]
                tunnel: [w486 _] -> w467
                frame #0 {
                  n127 = call "CS POLARIS BME DG.get i attribute.vi"("i ref in"=w480) -> ("i attribute"=w485:T10, "error out"=w479:errorcluster)  [unwired: 16 in, 1 out]
                  n128 = Unbundle By Name(w485) -> ("DIMLockedBy"=w484:i32)
                  n129 = call "ReleaseControl.vi"("error in (no error)"=w489, "locked by"=w487, "BME_DG_System in"=w491) -> ("error out"=w488:errorcluster, "locked by out"=w478:string, "BME_DG_System out"=w490:refnum<class "BME_DG_System.lvclass">)  [unwired: 4 in, 2 out]
                  n130 = call "UtilityLib.align string.vi"("stringIn"=w478, "error in (no error)"=w479) -> ("stringOut"=w483:string, "error out"=w482:errorcluster)  [unwired: 16 in]
                  n131 = call "CS POLARIS BME DG.CheckIn DG_System.vi"("error in"=w489, "timeout in ms (-1)"=w494, "BME_DG_System"=w490, "i ref in"=w480) -> ("error in"=w493:errorcluster, "i ref out"=w495:refnum<vi>)  [unwired: 5 in]
                  n132 = call "LVDimInterface.dis_update_service.vi"("my_serviceID"=w484, "data"=w483, "error in (no error)"=w482) -> ("error out"=w481:errorcluster)  [unwired: 14 in, 2 out]
                  n133 = call-poly "CoreLib.data 2 byte array.vi"("string"=w478) -> ("byteArray out"=w486:T1)  [unwired: 18 in]
                  n134 = call "UtilityLib.merge errors.vi"("error2 (no error)"=w488, "error1 (no error)"=w493) -> ("error out"=w492:errorcluster)
                  n135 = call <vilib>:"Clear Errors.vi"("error in (no error)"=w481) -> ()  [unwired: 6 in, 1 out]
                }
                frame #1 {
                }
              }
            }
            frame #1 {
              n136 = call "CoreLib.set data type mismatch.vi"("error in (no error)"=w500, "error source"=w498) -> ("error out"=w499:errorcluster)  [unwired: 17 in]
            }
          }
          n137 = call "BaseProcess.set event status.vi"("i ref in"=w464, "EventStatus"=w462, "error in (no error)"=w463) -> ("i ref out"=w461:refnum<vi>, "error out"=w457:errorcluster)  [unwired: 14 in, 1 out]
          n138 = call "CS POLARIS BME DG.Error2XMLFlatted call cluster.vi"("call cluster in"=w455, "byteArray in"=w453, "error in"=w457) -> ("call cluster out"=w454:T2, "error out"=w456:errorcluster)  [unwired: 7 in]
        }
        frame #8 {
          # "This is just an example. On how to use this VI. The names of the selector should be identical to the name of the corresponding event. Inside the false case, place the method you want to call."
          n139 = Unbundle By Name(w511) -> ("Data"=w515:T1)
          n140 = call-poly "CoreLib.byte array 2 data.vi"("byteArray"=w515) -> ("byteArray out"=w507:T1, "string"=w514:string, "error out"=w509:errorcluster)  [unwired: 16 in]
          n141 = call-poly "CoreLib.byte array 2 data.vi"("byteArray"=w507, "error in (no error)"=w509) -> ("string"=w506:string, "error out"=w508:errorcluster)  [unwired: 15 in, 1 out]
          n142 = case shown="No Error" w508 {
            tunnel: [w527 w554] -> w519
            tunnel: w521 -> [w529 w554]
            tunnel: w520 -> [w528 w553]
            tunnel: [w526 w552] -> w518
            tunnel: w517 -> [_ w551]
            tunnel: w514 -> [w525 _]
            tunnel: w506 -> [w524 _]
            tunnel: [w523 _] -> w505
            tunnel: [w522 _] -> w503
            frame #0 {
              w530 = 5000 ("timeout in ms (-1)")
              n143 = call "CS POLARIS BME DG.CheckOut DG_System.vi"("error IO"=w528, "timeout in ms (-1)"=w530, "i ref in"=w529) -> ("error out"=w533:errorcluster, "Q timed out"=w532:bool, "BME_DG_System out"=w534:refnum<class "BME_DG_System.lvclass">, "i ref out"=w531:refnum<vi>)  [unwired: 5 in]
              n144 = case "Time Out?" shown="False" w532 {
                tunnel: w534 -> [w543 _]
                tunnel: w533 -> [w542 w550]
                tunnel: [w544 w550] -> w526
                tunnel: [w548 w549] -> w527
                tunnel: w531 -> [w547 w549]
                tunnel: w530 -> [w546 _]
                tunnel: w525 -> [w540 _]
                tunnel: w524 -> [w539 _]
                tunnel: [w536 _] -> w523
                tunnel: [w535 _] -> w522
                frame #0 {
                  n145 = call "Check new DelayFormula and Update DelaysHW.vi"("Update HW?(false)"=FALSE, "error in (no error)"=w542, "Delay Formula"=w539, "ChnlName"=w540, "BME_DG_System in"=w543) -> ("error out"=w541:errorcluster, "Problem Chnls out"=w537:string[], "Abs. Delay"=w536:dbl)  [unwired: 3 in, 1 out]
                  n146 = Flatten To XML(anything=w537) -> (xml string=w535:string)
                  n147 = call "CS POLARIS BME DG.CheckIn DG_System.vi"("error in"=w542, "timeout in ms (-1)"=w546, "BME_DG_System"=w543, "i ref in"=w547) -> ("error in"=w545:errorcluster, "i ref out"=w548:refnum<vi>)  [unwired: 5 in]
                  n148 = call "UtilityLib.merge errors.vi"("error2 (no error)"=w541, "error1 (no error)"=w545) -> ("error out"=w544:errorcluster)
                }
                frame #1 {
                }
              }
            }
            frame #1 {
              n149 = call "CoreLib.set data type mismatch.vi"("error in (no error)"=w553, "error source"=w551) -> ("error out"=w552:errorcluster)  [unwired: 17 in]
            }
          }
          n150 = call-poly "CoreLib.data 2 byte array.vi"("f64"=w505) -> ("byteArray out"=w504:T1)  [unwired: 18 in]
          n151 = call "BaseProcess.set event status.vi"("i ref in"=w519, "EventStatus"=w517, "error in (no error)"=w518) -> ("i ref out"=w516:refnum<vi>, "error out"=w513:errorcluster)  [unwired: 14 in, 1 out]
          n152 = call-poly "CoreLib.data 2 byte array.vi"("byteArray"=w504, "string"=w503) -> ("byteArray out"=w502:T1)  [unwired: 17 in]
          n153 = call "CS POLARIS BME DG.Error2XMLFlatted call cluster.vi"("call cluster in"=w511, "byteArray in"=w502, "error in"=w513) -> ("call cluster out"=w510:T2, "error out"=w512:errorcluster)  [unwired: 7 in]
        }
        frame #9 {
          # "This is just an example. On how to use this VI. The names of the selector should be identical to the name of the corresponding event. Inside the false case, place the method you want to call."
          n154 = case shown="No Error" w555 {
            tunnel: [w568 w595] -> w564
            tunnel: w565 -> [w570 w595]
            tunnel: w555 -> [w569 w594]
            tunnel: [w567 w593] -> w563
            tunnel: w562 -> [_ w592]
            tunnel: [w566 _] -> w556
            frame #0 {
              w571 = 5000 ("timeout in ms (-1)")
              n155 = call "CS POLARIS BME DG.CheckOut DG_System.vi"("error IO"=w569, "timeout in ms (-1)"=w571, "i ref in"=w570) -> ("error out"=w574:errorcluster, "Q timed out"=w573:bool, "BME_DG_System out"=w575:refnum<class "BME_DG_System.lvclass">, "i ref out"=w572:refnum<vi>)  [unwired: 5 in]
              n156 = case "Time Out?" shown="False" w573 {
                tunnel: w575 -> [w583 _]
                tunnel: w574 -> [w582 w591]
                tunnel: [w585 w591] -> w567
                tunnel: [w589 w590] -> w568
                tunnel: w572 -> [w588 w590]
                tunnel: w571 -> [w587 _]
                tunnel: [w584 _] -> w566
                frame #0 {
                  n157 = call "Read System Name.vi"("error in (no error)"=w582, "BME_DG_System in"=w583) -> ("error out"=w579:errorcluster, "log Name"=w580:string, "BME_DG_System out"=w581:refnum<class "BME_DG_System.lvclass">)  [unwired: 7 in]
                  n158 = call "GFV DG Systems.vi"("BME_DG_System"=w581, "SystemlName"=w580, "error in"=w579) -> ("ChnlNames"=w576:string[], "error out"=w578:errorcluster)  [unwired: 7 in, 4 out]
                  n159 = call "CS POLARIS BME DG.CheckIn DG_System.vi"("error in"=w582, "timeout in ms (-1)"=w587, "BME_DG_System"=w581, "i ref in"=w588) -> ("error in"=w586:errorcluster, "i ref out"=w589:refnum<vi>)  [unwired: 5 in]
                  n160 = Flatten To XML(anything=w576) -> (xml string=w577:string)
                  n161 = call "UtilityLib.merge errors.vi"("error2 (no error)"=w578, "error1 (no error)"=w586) -> ("error out"=w585:errorcluster)
                  n162 = call-poly "CoreLib.data 2 byte array.vi"("string"=w577) -> ("byteArray out"=w584:T1)  [unwired: 18 in]
                }
                frame #1 {
                }
              }
            }
            frame #1 {
              n163 = call "CoreLib.set data type mismatch.vi"("error in (no error)"=w594, "error source"=w592) -> ("error out"=w593:errorcluster)  [unwired: 17 in]
            }
          }
          n164 = call "BaseProcess.set event status.vi"("i ref in"=w564, "EventStatus"=w562, "error in (no error)"=w563) -> ("i ref out"=w561:refnum<vi>, "error out"=w560:errorcluster)  [unwired: 14 in, 1 out]
          n165 = call "CS POLARIS BME DG.Error2XMLFlatted call cluster.vi"("call cluster in"=w558, "byteArray in"=w556, "error in"=w560) -> ("call cluster out"=w557:T2, "error out"=w559:errorcluster)  [unwired: 7 in]
        }
      }
    }
    frame #1 {
    }
  }
  "answer cluster" <- w7
  "i ref out" <- w3
  "error out" <- w2
